vi "Read String Var.vi"(2 "错误输入（无错误）":errorcluster, 3 "Tag IN":string, 4 "Ds PLCTags IN":T1[](array[typedef])) -> (0 "error out":errorcluster, 1 "String Var out":string)   [LabVIEW 2014]
uses:
  DataSocket_Tags.ctl
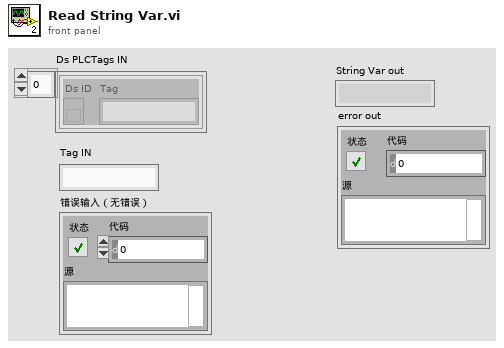
[diagram p1: front panel]
types:
  T1 = typedef "DataSocket_Tags.ctl" = cluster{"Ds ID":refnum<k13>, "Tag":string}
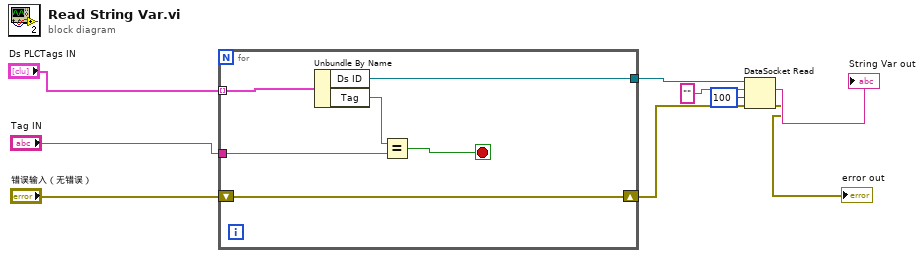
[diagram p0: block diagram]
diagram:
  n1 = for {
    tunnel: "Ds PLCTags IN" -> [w15] mode=indexing
    tunnel: "Tag IN" -> [w13]
    tunnel: [w11] -> w4
    shift-right: [w10] -> w3
    shift-left: "错误输入（无错误）" -> [w10]
    stop <- w12 stop-if-true
    n2 = Unbundle By Name(w15) -> ("Ds ID"=w11:refnum<k13>, "Tag"=w14:string)
    n3 = Equal?(x=w14, y=w13) -> (x = y?=w12:bool)
  }
  n4 = DataSocket Read(8:w3, 9:100 ("毫秒超时(10000)"), 10:"", 11:w4) -> (0:→"error out":errorcluster, 2:→"String Var out":string)  [unwired: 1 in, 5 out]
